vi "Interrogate Target.vi"(8 "Error In":errorcluster, 11 "Install LV Data":T1={"SSH Session"=refnum, "Status Log"="", "Detailed Log"="", "Credentials"={"Hostname or IP"="192.168.7.2", "Username"="root", "Password"=""}, "Target Info"={"OS Version"="", "CPU"="", "Systemd Version"="", "Internet Access"=FALSE, "Device Type"="", "LV Installed Ver"="", "LV Available Ver"="", "LV Upgrade Available"=FALSE, "Hostname"="", "NIC Info"=[]}, "Reboot Required?"=FALSE}) -> (0 "Error Out":errorcluster, 1 "Status":string="Unable To Interrogate The Device", 2 "Target Info":T2, 3 "Install LV Data":T1={"SSH Session"=refnum, "Status Log"="", "Detailed Log"="", "Credentials"={"Hostname or IP"="192.168.7.2", "Username"="root", "Password"=""}, "Target Info"={"OS Version"="", "CPU"="", "Systemd Version"="", "Internet Access"=FALSE, "Device Type"="", "LV Installed Ver"="", "LV Available Ver"="", "LV Upgrade Available"=FALSE, "Hostname"="", "NIC Info"=[]}, "Reboot Required?"=FALSE})   [LabVIEW 2020, in "LMH-LINX.lvlib"]
uses:
  LMH-LINX.lvlib
  Target Info.ctl
  NIC Info.ctl
  NIC Mode.ctl
  Install LV Data.ctl
  Generic FGV State.ctl
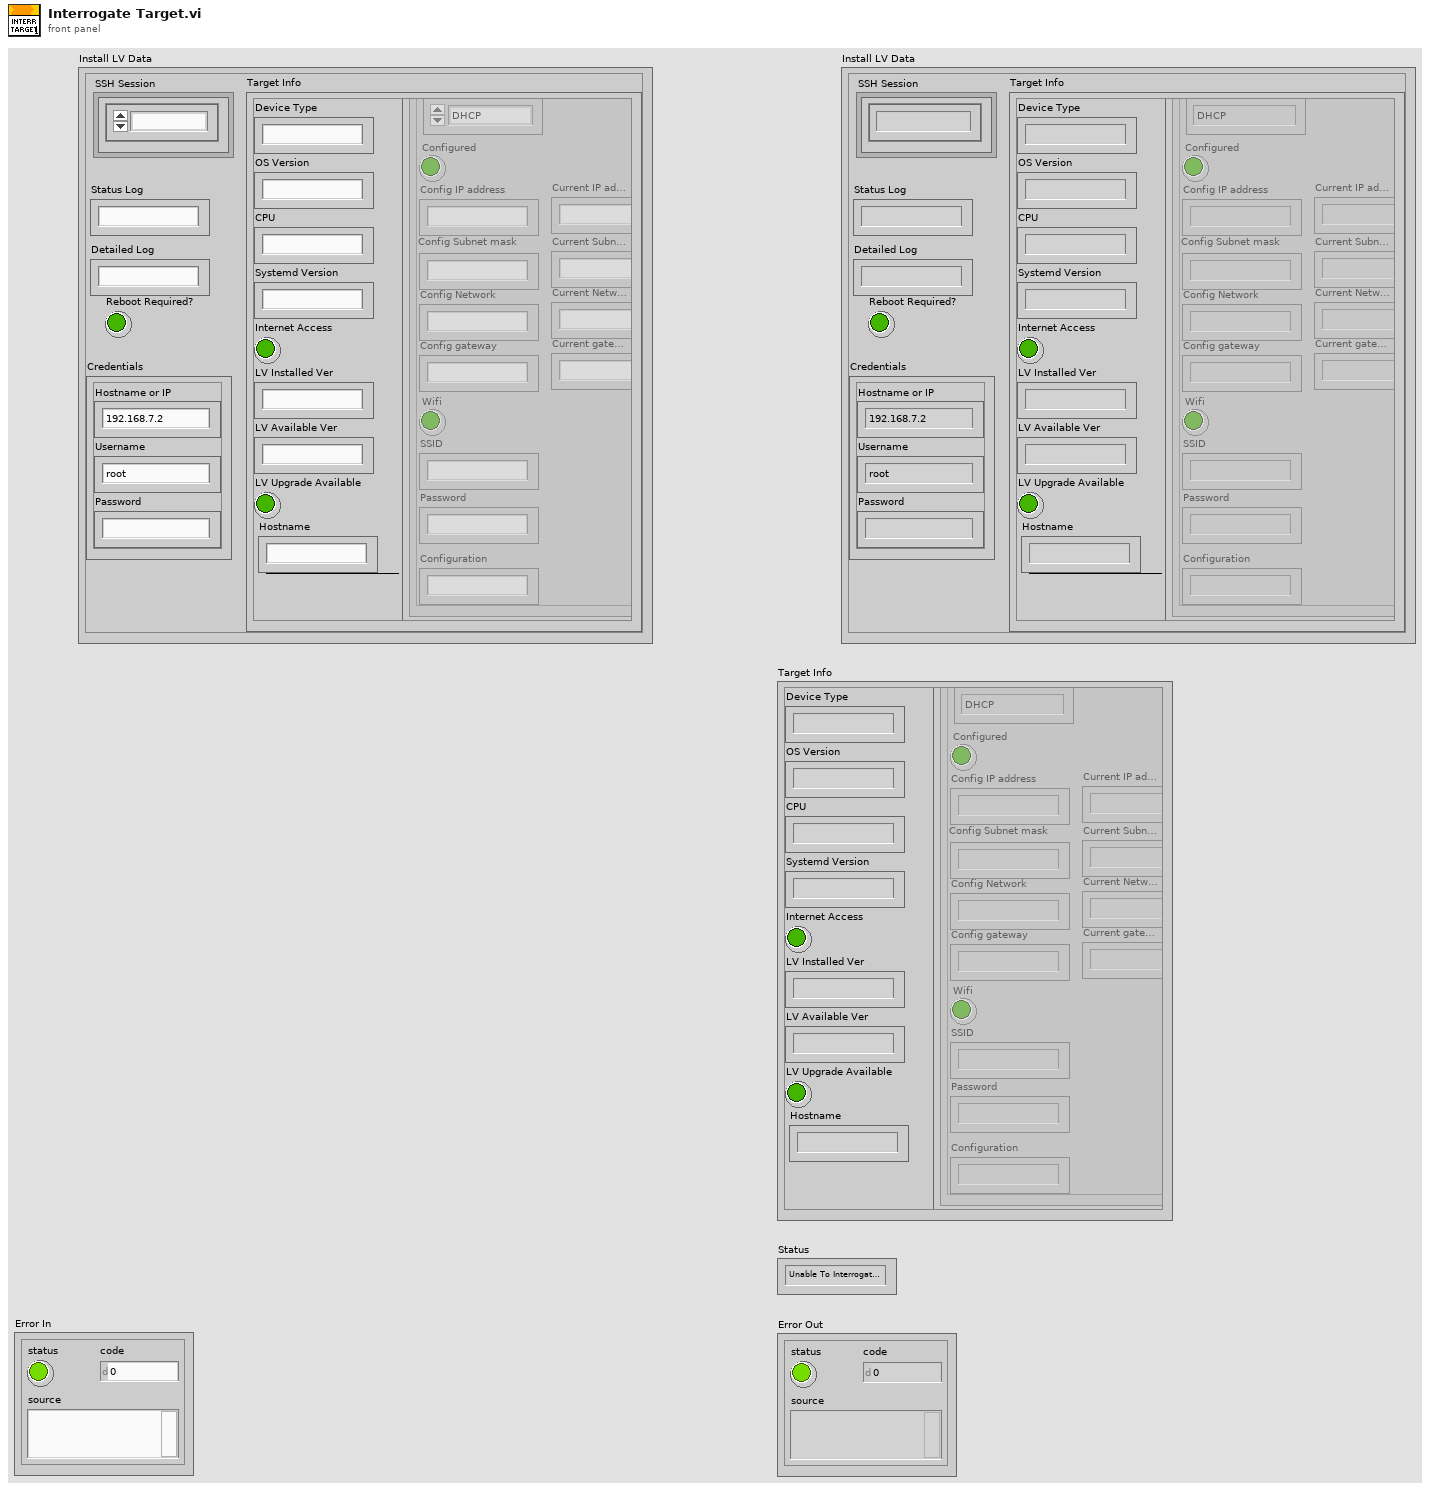
[diagram p1: front panel]
types:
  T1 = typedef "LMH-LINX.lvlib/Install LV Data.ctl" = cluster{"SSH Session":refnum<k1>, "Status Log":string, "Detailed Log":string, "Credentials":cluster{"Hostname or IP":string, "Username":string, "Password":string}, "Target Info":T2, "Reboot Required?":bool}
  T2 = typedef "LMH-LINX.lvlib/Target Info.ctl" = cluster{"OS Version":string, "CPU":string, "Systemd Version":string, "Internet Access":bool, "Device Type":string, "LV Installed Ver":string, "LV Available Ver":string, "LV Upgrade Available":bool, "Hostname":string, "NIC Info":T3[]}
  T3 = typedef "LMH-LINX.lvlib/NIC Info.ctl" = cluster{"Name":string, "NIC Mode":T4, "Configured":bool, "Config IP address":string, "Config Subnet mask":string, "Config Network":string, "Config gateway":string, "Wifi":bool, "SSID":string, "Password":string, "Configuration":string, "Current IP address":string, "Current Subnet mask":string, "Current gateway":string, "Current Network":string}
  T4 = typedef "LMH-LINX.lvlib/NIC Mode.ctl" = enum16{"DHCP", "Static", "Loopback"}
  T5 = typedef "LMH-LINX.lvlib/Generic FGV State.ctl" = enum16{"Get", "Set"}
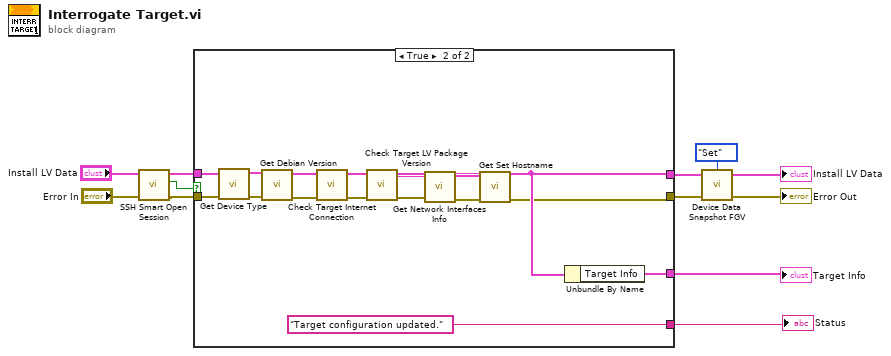
[diagram p0: block diagram]
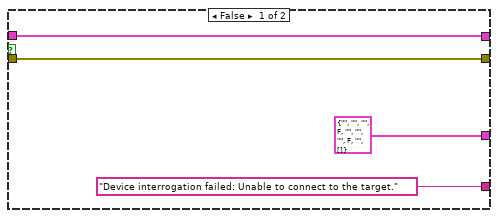
[diagram p2: hidden frame]
diagram:
  n1 = call "SSH Smart Open Session.vi"("Error In"="Error In", "Install LV Data in"="Install LV Data") -> ("Error Out"=w7:errorcluster, "Connected?"=w5:bool, "Install LV Data out"=w8:T1)  [unwired: 6 in, 1 out]
  n2 = case shown="True" w5 {
    tunnel: [T2 {"OS Version"="", "CPU"="", "Systemd Version"="", "Internet Access"=FALSE, "Device Type"="", "LV Installed Ver"="", "LV Available Ver"="", "LV Upgrade Available"=FALSE, "Hostname"="", "NIC Info"=[]} ("Target Info") w26] -> w11
    tunnel: [w13 w18] -> w4
    tunnel: w7 -> [w13 w16]
    tunnel: ["Device interrogation failed: Unable to connect to the target." "Target configuration updated."] -> w10
    tunnel: w8 -> [w12 w17]
    tunnel: [w12 w19] -> w3
    frame False {
    }
    frame True {
      n3 = call "Get Device Type.vi"("Error In"=w16, "Install LV Data"=w17) -> ("Error Out"=w31:errorcluster, "Install LV Data"=w29:T1)  [unwired: 7 in, 1 out]
      n4 = call "Get Debian Version.vi"("Error In"=w31, "Install LV Data"=w29) -> ("Error Out"=w27:errorcluster, "Install LV Data"=w28:T1)  [unwired: 7 in, 1 out]
      n5 = call "Check Target Internet Connection.vi"("Error In"=w27, "Install LV Data"=w28) -> ("Error Out"=w24:errorcluster, "Install LV Data"=w25:T1)  [unwired: 8 in]
      n6 = call "Check Target LV Package Version.vi"("Error In"=w24, "Install LV Data"=w25) -> ("Error Out"=w22:errorcluster, "Install LV Data"=w23:T1)  [unwired: 5 in, 3 out]
      n7 = call "Get Network Interfaces Info.vi"("Error In"=w22, "Install LV Data"=w23) -> ("Error Out"=w20:errorcluster, "Install LV Data"=w21:T1)  [unwired: 8 in]
      n8 = call "Get Set Hostname.vi"("Error In"=w20, "Install LV Data"=w21) -> ("Error Out"=w18:errorcluster, "Install LV Data"=w19:T1)  [unwired: 7 in, 1 out]
      n9 = Unbundle By Name(w19) -> ("Target Info"=w26:T2)
    }
  }
  "Error Out" <- w4
  "Target Info" <- w11
  "Status" <- w10
  n10 = call "Device Data Snapshot FGV.vi"("Install LV Data"=w3, "FGV State"=Generic_FGV_State."Set") -> ("Install LV Data"=→"Install LV Data":T1)  [unwired: 2 in]
